vi "Blinking LED.vi"() -> ()   [LabVIEW 2019]
panel:
  in  "Number of flashes":dbl
  in  "Frequency 2":dbl
  out "My LED":bool
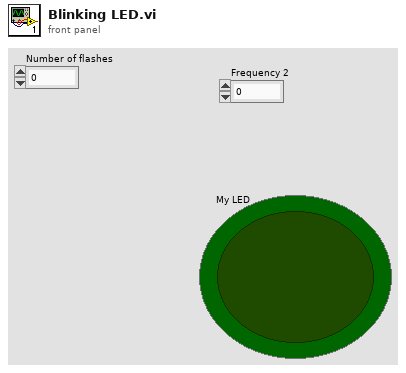
[diagram p1: front panel]
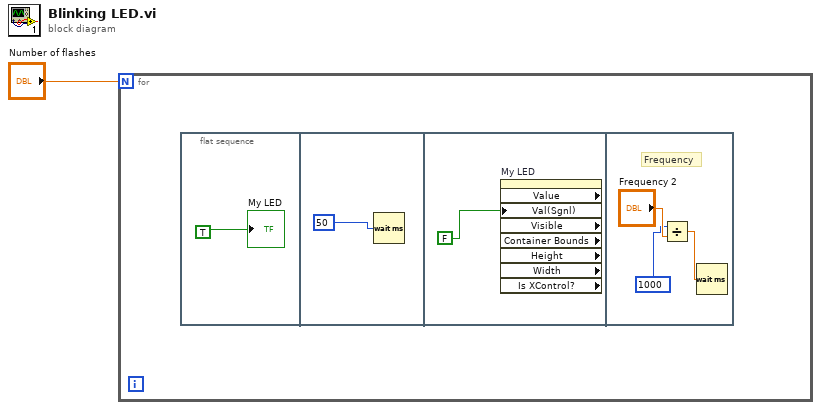
[diagram p0: block diagram]
diagram:
  n1 = for {
    N: "Number of flashes" -> [_]
    n2 = flat-sequence {
      frame #0 {
        "My LED" <- TRUE
      }
      frame #1 {
        n3 = Wait (ms)(milliseconds to wait=50) -> ()  [unwired: 1 out]
      }
      frame #2 {
        n4 = property on="My LED" class="Bool (strict)" props=["Value", "Val(Sgnl)", "Visible", "Container Bounds", "Height", "Width", "Is XControl?"]("Val(Sgnl)"=FALSE) -> ()  [unwired: 2 in, 8 out]
      }
      frame #3 {
        # "Frequency"
        n5 = Divide(x=1000, y="Frequency 2") -> (x/y=w7:dbl)
        n6 = Wait (ms)(milliseconds to wait=w7) -> ()  [unwired: 1 out]
      }
    }
  }
